vi "loop error, restart vi_polymorphic.vi"   [LabVIEW 2013]
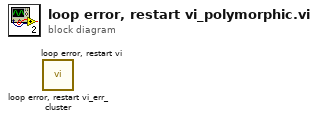
[diagram p0: block diagram]
diagram:
  n1 = call "loop error, restart vi_err_cluster.vi"() -> ()  [unwired: 12 in]
  n2 = call "loop error, restart vi.vi"() -> ()  [unwired: 12 in]
